vi "Get panel triangle edge link indices.vi"(1 "Panel triangles in":T1[](array[typedef])) -> (0 "Panel triangles out":T1[](array[typedef]))   [LabVIEW 2017]
uses:
  ctls/Triangle panel.ctl
  Dot product_3Dpf.vi
panel:
  out "Progress":i32(slide) scale=0.0..3330.0
  out "N panels":i32
  out "Panel number":i32
  # "Computing panel links (needed for sfc. gradient & Cp calcs.)"
  # "of"
  # "PN 23/10/17"
  # "Vertices"
  # "Edges"
  # "Unit normal"
  # "Control point"
  # "Edge\nlinks \n(tri index)"
  # "Vertices"
  # "Edges"
  # "Unit normal"
  # "Control point"
  # "Edge\nlinks \n(tri index)"
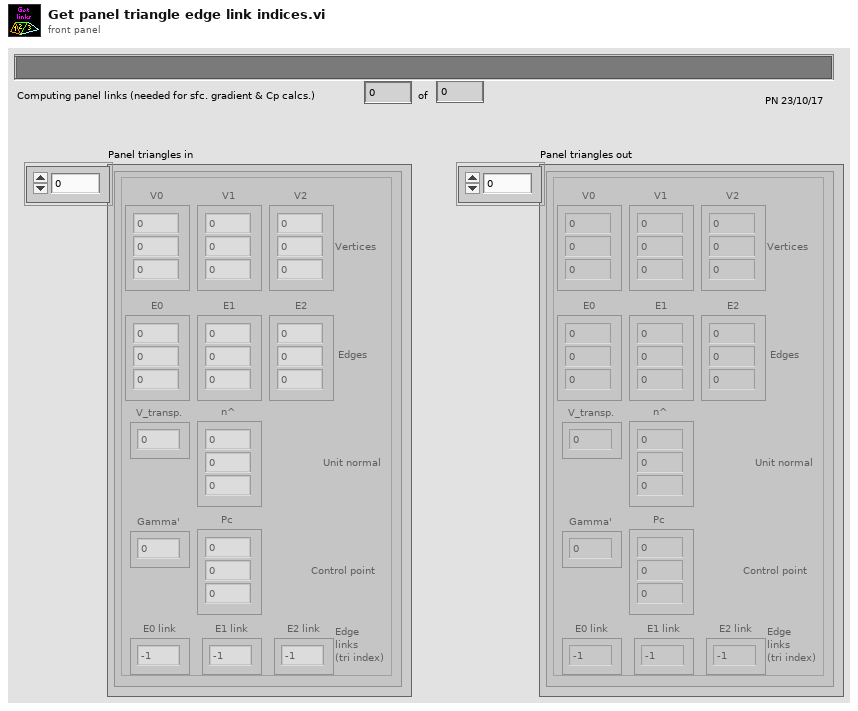
[diagram p1: front panel]
types:
  T1 = typedef "Triangle panel.ctl" = cluster{"V0":sgl[], "V1":sgl[], "V2":sgl[], "E0":sgl[], "E1":sgl[], "E2":sgl[], "n^":sgl[], "Pc":sgl[], "Gamma'":sgl, "V_transp.":sgl, "E0 link":i32, "E1 link":i32, "E2 link":i32}
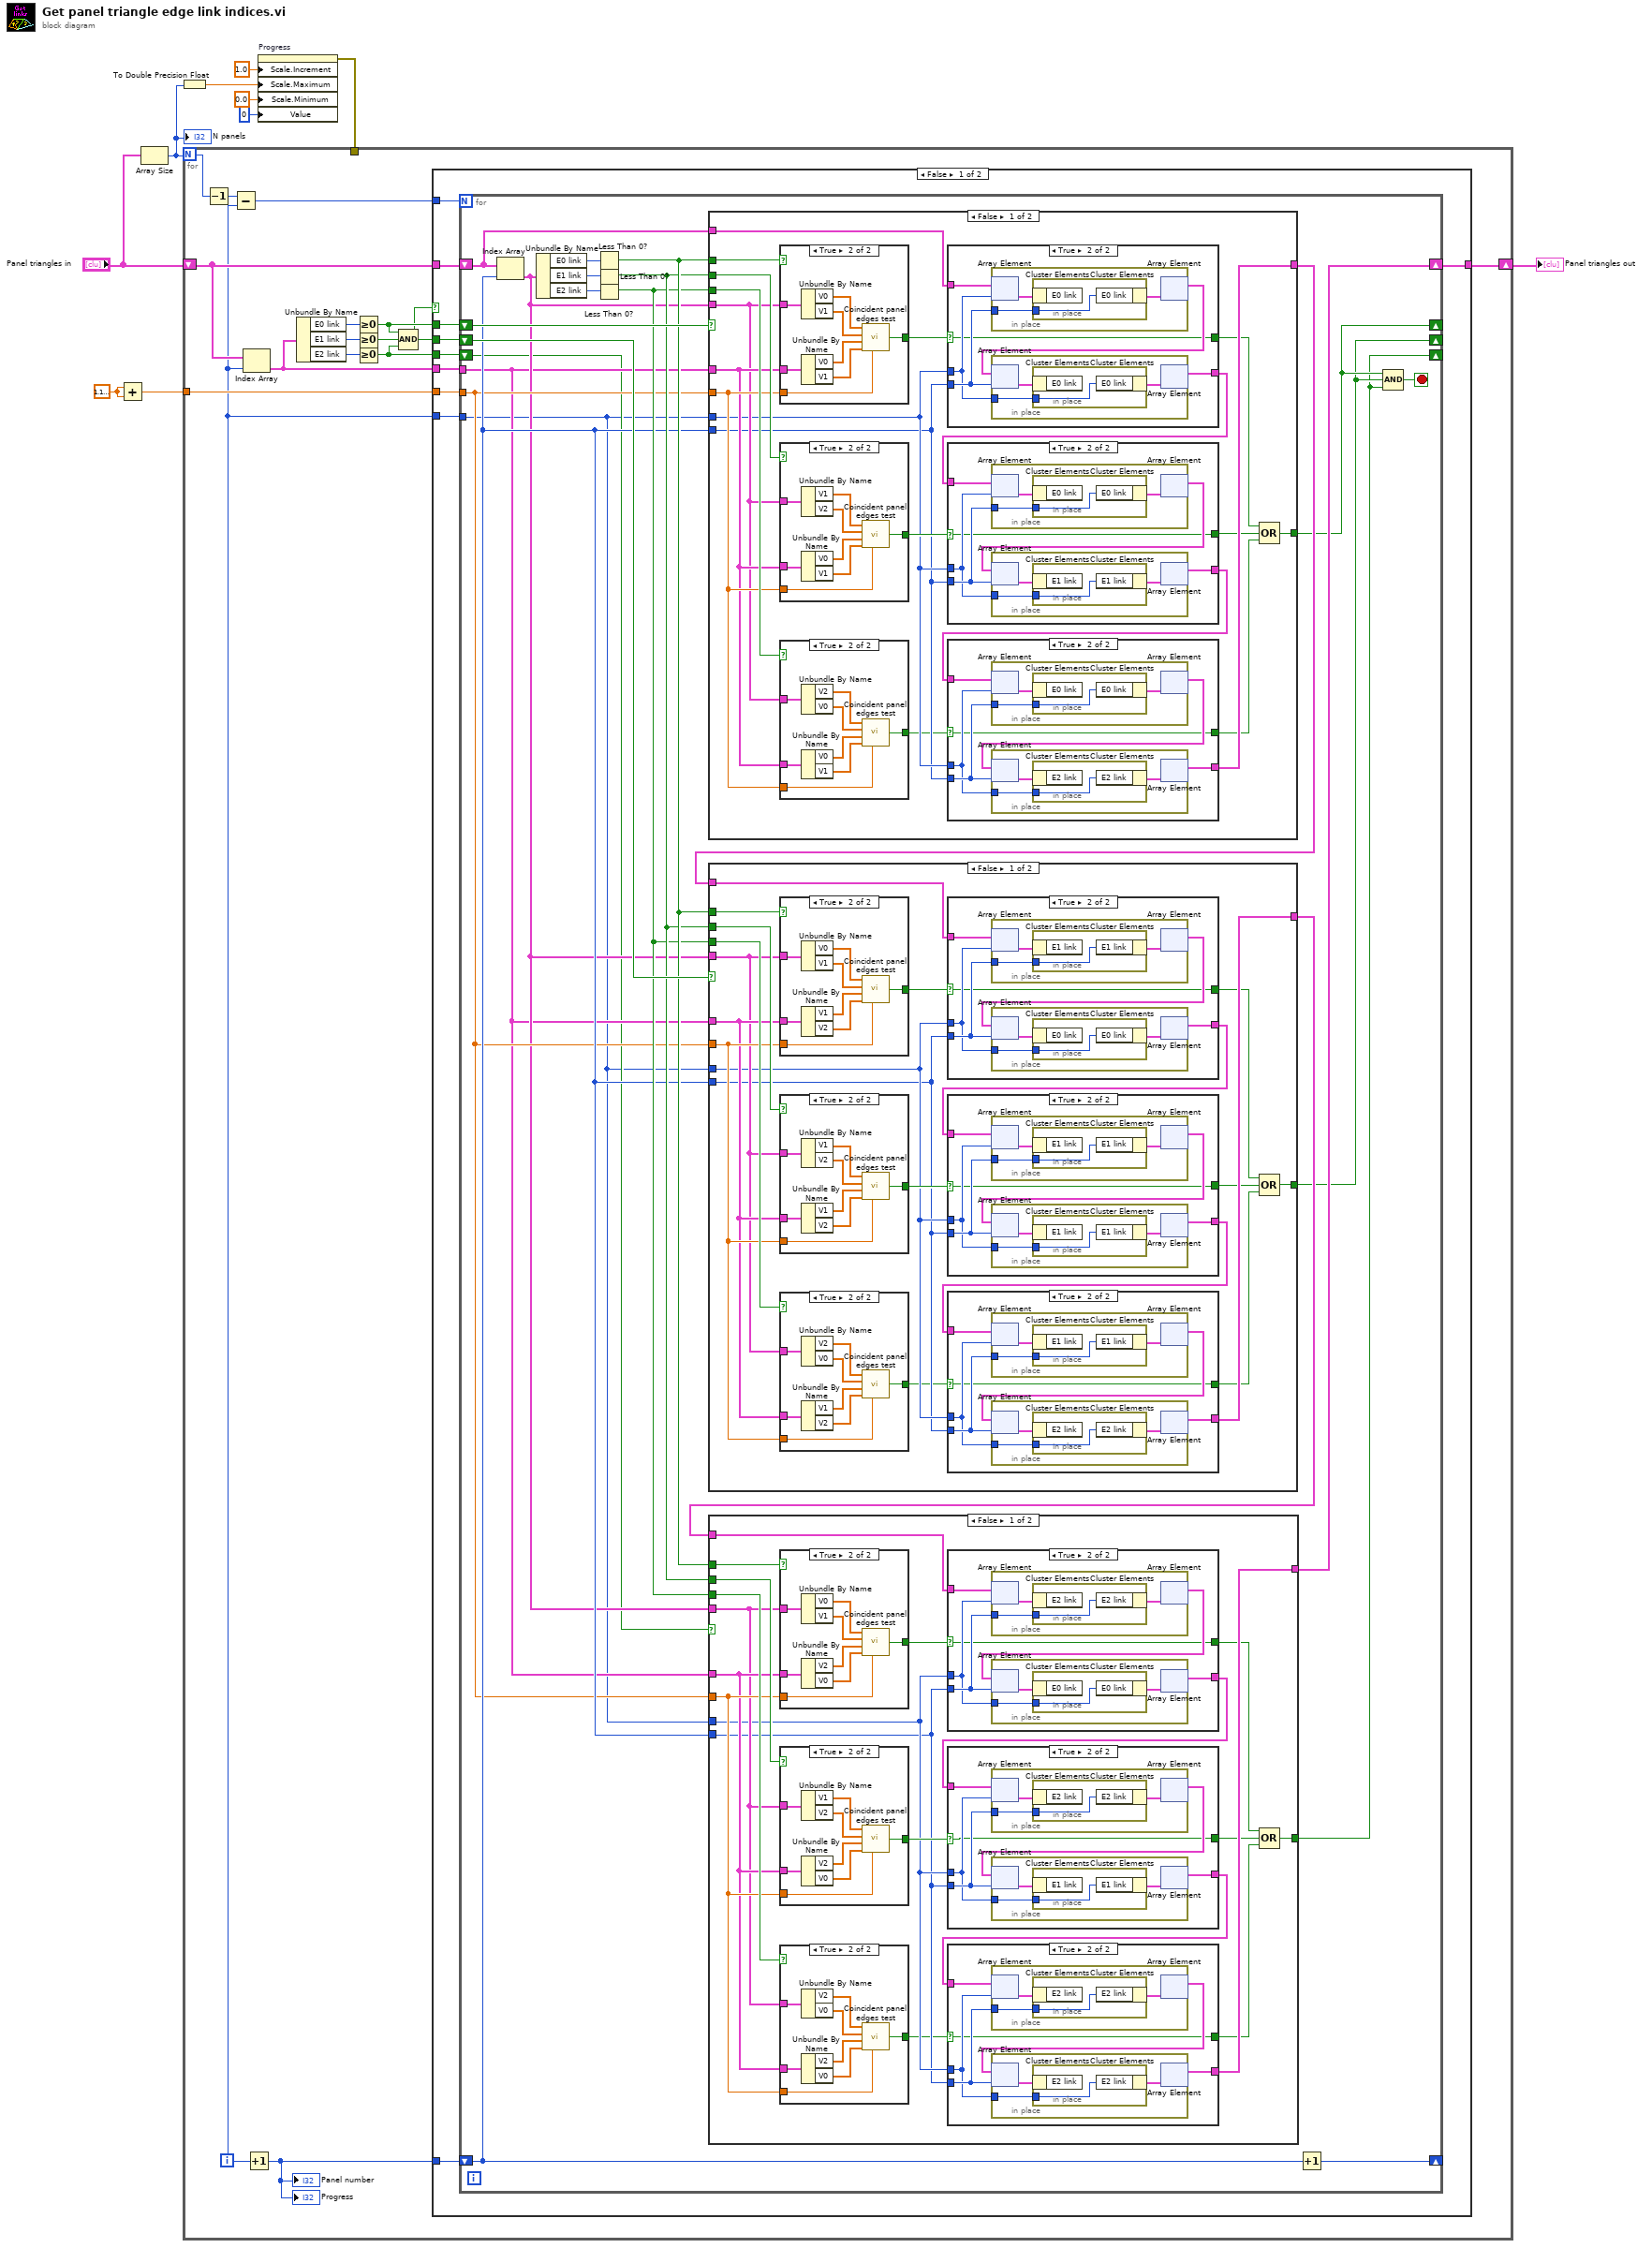
[diagram p0: block diagram]
diagram:
  w2 = sgl 1.1920929e-07
  n1 = Add(x=w2, y=w2) -> (x+y=w3:sgl)
  n2 = Array Size(array="Panel triangles in") -> (size(s)=w6:i32)
  "N panels" <- w6
  n3 = To Double Precision Float(number=w6) -> (double precision float=w1:dbl)
  n4 = property on="Progress" class="Slide (strict)"("Scale.Increment"=1.0 ("Scale.Range:Increment"), "Scale.Maximum"=w1, "Scale.Minimum"=0.0 ("Scale.Range:Minimum"), "Value"=0 ("Progress")) -> (error out=w4:errorcluster)  [unwired: 2 in, 1 out]
  n5 = for {
    N: w6 -> [w26]
    shift-right: [w12] -> w9
    shift-left: "Panel triangles in" -> [w16]
    tunnel: w3 -> [w14]
    tunnel: w4 -> [_]
    i -> [w13]
    n6 = Decrement(x=w26) -> (x-1=w25:i32)
    n7 = Subtract(x=w25, y=w13) -> (x-y=w24:i32)
    n8 = Index Array(array=w16, index=w13) -> (element=w15:T1)
    n9 = Increment(x=w13) -> (x+1=w11:i32)
    "Panel number" <- w11
    "Progress" <- w11
    n10 = Unbundle By Name(w15) -> ("E0 link"=w21:i32, "E1 link"=w22:i32, "E2 link"=w23:i32)
    n11 = Greater Or Equal To 0?(x=w21) -> (x >= 0?=w20:bool)
    n12 = Greater Or Equal To 0?(x=w22) -> (x >= 0?=w19:bool)
    n13 = Greater Or Equal To 0?(x=w23) -> (x >= 0?=w18:bool)
    n14 = Compound Arithmetic op=AND(w20, w19, w18) -> (w17:bool)
    n15 = case shown="False" w17 {
      tunnel: w24 -> [w36 _]
      tunnel: w11 -> [w35 _]
      tunnel: w16 -> [w34 w348]
      tunnel: w20 -> [w33 _]
      tunnel: w19 -> [w32 _]
      tunnel: w18 -> [w31 _]
      tunnel: w15 -> [w30 _]
      tunnel: w14 -> [w29 _]
      tunnel: w13 -> [w28 _]
      tunnel: [w27 w348] -> w12
      frame False {
        n16 = for {
          N: w36 -> [_]
          shift-right: [w59] -> _
          shift-left: w35 -> [w49]
          tunnel: w30 -> [w46]
          shift-right: [w44] -> w27
          shift-left: w34 -> [w53]
          tunnel: w29 -> [w48]
          tunnel: w28 -> [w43]
          shift-right: [w39] -> _
          shift-left: w33 -> [w55]
          shift-right: [w38] -> _
          shift-left: w32 -> [w54]
          shift-right: [w37] -> _
          shift-left: w31 -> [w45]
          stop <- w42 stop-if-true
          n17 = Index Array(array=w53, index=w49) -> (element=w47:T1)
          n18 = Unbundle By Name(w47) -> ("E0 link"=w56:i32, "E1 link"=w57:i32, "E2 link"=w58:i32)
          n19 = Less Than 0?(x=w56) -> (x < 0?=w52:bool)
          n20 = Less Than 0?(x=w57) -> (x < 0?=w51:bool)
          n21 = Less Than 0?(x=w58) -> (x < 0?=w50:bool)
          n22 = case shown="False" w55 {
            selector: w55 -> [_ w346]
            tunnel: w52 -> [w270 _]
            tunnel: w51 -> [w269 _]
            tunnel: w50 -> [w268 _]
            tunnel: w47 -> [w265 _]
            tunnel: w46 -> [w266 _]
            tunnel: w48 -> [w267 _]
            tunnel: w53 -> [w263 w347]
            tunnel: w43 -> [w259 _]
            tunnel: w49 -> [w258 _]
            tunnel: [w256 w347] -> w41
            tunnel: [w252 w346] -> w39
            frame False {
              n23 = case shown="True" w270 {
                selector: w270 -> [w337 _]
                tunnel: w265 -> [_ w345]
                tunnel: w266 -> [_ w344]
                tunnel: w267 -> [_ w339]
                tunnel: [w337 w338] -> w264
                frame False {
                }
                frame True {
                  n24 = Unbundle By Name(w345) -> ("V0"=w343:sgl[], "V1"=w342:sgl[])
                  n25 = Unbundle By Name(w344) -> ("V0"=w341:sgl[], "V1"=w340:sgl[])
                  n26 = call "Coincident panel edges test.vi"("epsilon"=w339, "V1_1"=w340, "V1_0"=w341, "V0_1"=w342, "V0_0"=w343) -> ("Edges are coincident"=w338:bool)  [unwired: 1 in]
                }
              }
              n27 = case shown="True" w269 {
                selector: w269 -> [w328 _]
                tunnel: w265 -> [_ w336]
                tunnel: w266 -> [_ w335]
                tunnel: w267 -> [_ w330]
                tunnel: [w328 w329] -> w261
                frame False {
                }
                frame True {
                  n28 = Unbundle By Name(w336) -> ("V1"=w334:sgl[], "V2"=w333:sgl[])
                  n29 = Unbundle By Name(w335) -> ("V0"=w332:sgl[], "V1"=w331:sgl[])
                  n30 = call "Coincident panel edges test.vi"("epsilon"=w330, "V1_1"=w331, "V1_0"=w332, "V0_1"=w333, "V0_0"=w334) -> ("Edges are coincident"=w329:bool)  [unwired: 1 in]
                }
              }
              n31 = case shown="True" w268 {
                selector: w268 -> [w319 _]
                tunnel: w265 -> [_ w327]
                tunnel: w266 -> [_ w326]
                tunnel: w267 -> [_ w321]
                tunnel: [w319 w320] -> w257
                frame False {
                }
                frame True {
                  n32 = Unbundle By Name(w327) -> ("V2"=w325:sgl[], "V0"=w324:sgl[])
                  n33 = Unbundle By Name(w326) -> ("V0"=w323:sgl[], "V1"=w322:sgl[])
                  n34 = call "Coincident panel edges test.vi"("epsilon"=w321, "V1_1"=w322, "V1_0"=w323, "V0_1"=w324, "V0_0"=w325) -> ("Edges are coincident"=w320:bool)  [unwired: 1 in]
                }
              }
              n35 = case shown="True" w264 {
                selector: w264 -> [w303 w305]
                tunnel: w263 -> [w304 w310]
                tunnel: w259 -> [_ w307]
                tunnel: w258 -> [_ w308]
                tunnel: [w304 w306] -> w262
                tunnel: [w303 w305] -> w254
                frame False {
                }
                frame True {
                  n36 = in-place {
                    in-place-border: w308 -> [w316]
                    n37 = in-place-array #1(w310, w307) -> (w317:T1)
                    n38 = in-place {
                      in-place-border: w316 -> [w318]
                      n39 = in-place-cluster #2(w317) -> ()  [unwired: 1 out]
                      n40 = in-place-cluster #2("E0 link"=w318) -> (w315:T1)
                    }
                    n41 = in-place-array #1(w315) -> (w309:T1[])  [unwired: 1 out]
                  }
                  n42 = in-place {
                    in-place-border: w307 -> [w312]
                    n43 = in-place-array #3(w309, w308) -> (w313:T1)
                    n44 = in-place {
                      in-place-border: w312 -> [w314]
                      n45 = in-place-cluster #4(w313) -> ()  [unwired: 1 out]
                      n46 = in-place-cluster #4("E0 link"=w314) -> (w311:T1)
                    }
                    n47 = in-place-array #3(w311) -> (w306:T1[])  [unwired: 1 out]
                  }
                }
              }
              n48 = case shown="True" w261 {
                selector: w261 -> [w287 w289]
                tunnel: w262 -> [w288 w294]
                tunnel: w259 -> [_ w291]
                tunnel: w258 -> [_ w292]
                tunnel: [w288 w290] -> w260
                tunnel: [w287 w289] -> w255
                frame False {
                }
                frame True {
                  n49 = in-place {
                    in-place-border: w292 -> [w300]
                    n50 = in-place-array #5(w294, w291) -> (w301:T1)
                    n51 = in-place {
                      in-place-border: w300 -> [w302]
                      n52 = in-place-cluster #6(w301) -> ()  [unwired: 1 out]
                      n53 = in-place-cluster #6("E0 link"=w302) -> (w299:T1)
                    }
                    n54 = in-place-array #5(w299) -> (w293:T1[])  [unwired: 1 out]
                  }
                  n55 = in-place {
                    in-place-border: w291 -> [w296]
                    n56 = in-place-array #7(w293, w292) -> (w297:T1)
                    n57 = in-place {
                      in-place-border: w296 -> [w298]
                      n58 = in-place-cluster #8(w297) -> ()  [unwired: 1 out]
                      n59 = in-place-cluster #8("E1 link"=w298) -> (w295:T1)
                    }
                    n60 = in-place-array #7(w295) -> (w290:T1[])  [unwired: 1 out]
                  }
                }
              }
              n61 = case shown="True" w257 {
                selector: w257 -> [w271 w273]
                tunnel: w260 -> [w272 w278]
                tunnel: w259 -> [_ w275]
                tunnel: w258 -> [_ w276]
                tunnel: [w272 w274] -> w256
                tunnel: [w271 w273] -> w253
                frame False {
                }
                frame True {
                  n62 = in-place {
                    in-place-border: w276 -> [w284]
                    n63 = in-place-array #9(w278, w275) -> (w285:T1)
                    n64 = in-place {
                      in-place-border: w284 -> [w286]
                      n65 = in-place-cluster #10(w285) -> ()  [unwired: 1 out]
                      n66 = in-place-cluster #10("E0 link"=w286) -> (w283:T1)
                    }
                    n67 = in-place-array #9(w283) -> (w277:T1[])  [unwired: 1 out]
                  }
                  n68 = in-place {
                    in-place-border: w275 -> [w280]
                    n69 = in-place-array #11(w277, w276) -> (w281:T1)
                    n70 = in-place {
                      in-place-border: w280 -> [w282]
                      n71 = in-place-cluster #12(w281) -> ()  [unwired: 1 out]
                      n72 = in-place-cluster #12("E2 link"=w282) -> (w279:T1)
                    }
                    n73 = in-place-array #11(w279) -> (w274:T1[])  [unwired: 1 out]
                  }
                }
              }
              n74 = Compound Arithmetic op=OR(w254, w255, w253) -> (w252:bool)
            }
            frame True {
            }
          }
          n75 = case shown="False" w54 {
            selector: w54 -> [_ w250]
            tunnel: w52 -> [w174 _]
            tunnel: w51 -> [w173 _]
            tunnel: w50 -> [w172 _]
            tunnel: w47 -> [w169 _]
            tunnel: w46 -> [w170 _]
            tunnel: w48 -> [w171 _]
            tunnel: w41 -> [w167 w251]
            tunnel: w43 -> [w163 _]
            tunnel: w49 -> [w162 _]
            tunnel: [w160 w251] -> w40
            tunnel: [w156 w250] -> w38
            frame False {
              n76 = case shown="True" w174 {
                selector: w174 -> [w241 _]
                tunnel: w169 -> [_ w249]
                tunnel: w170 -> [_ w248]
                tunnel: w171 -> [_ w243]
                tunnel: [w241 w242] -> w168
                frame False {
                }
                frame True {
                  n77 = Unbundle By Name(w249) -> ("V0"=w247:sgl[], "V1"=w246:sgl[])
                  n78 = Unbundle By Name(w248) -> ("V1"=w245:sgl[], "V2"=w244:sgl[])
                  n79 = call "Coincident panel edges test.vi"("epsilon"=w243, "V1_1"=w244, "V1_0"=w245, "V0_1"=w246, "V0_0"=w247) -> ("Edges are coincident"=w242:bool)  [unwired: 1 in]
                }
              }
              n80 = case shown="True" w173 {
                selector: w173 -> [w232 _]
                tunnel: w169 -> [_ w240]
                tunnel: w170 -> [_ w239]
                tunnel: w171 -> [_ w234]
                tunnel: [w232 w233] -> w165
                frame False {
                }
                frame True {
                  n81 = Unbundle By Name(w240) -> ("V1"=w238:sgl[], "V2"=w237:sgl[])
                  n82 = Unbundle By Name(w239) -> ("V1"=w236:sgl[], "V2"=w235:sgl[])
                  n83 = call "Coincident panel edges test.vi"("epsilon"=w234, "V1_1"=w235, "V1_0"=w236, "V0_1"=w237, "V0_0"=w238) -> ("Edges are coincident"=w233:bool)  [unwired: 1 in]
                }
              }
              n84 = case shown="True" w172 {
                selector: w172 -> [w223 _]
                tunnel: w169 -> [_ w231]
                tunnel: w170 -> [_ w230]
                tunnel: w171 -> [_ w225]
                tunnel: [w223 w224] -> w161
                frame False {
                }
                frame True {
                  n85 = Unbundle By Name(w231) -> ("V2"=w229:sgl[], "V0"=w228:sgl[])
                  n86 = Unbundle By Name(w230) -> ("V1"=w227:sgl[], "V2"=w226:sgl[])
                  n87 = call "Coincident panel edges test.vi"("epsilon"=w225, "V1_1"=w226, "V1_0"=w227, "V0_1"=w228, "V0_0"=w229) -> ("Edges are coincident"=w224:bool)  [unwired: 1 in]
                }
              }
              n88 = case shown="True" w168 {
                selector: w168 -> [w207 w209]
                tunnel: w167 -> [w208 w214]
                tunnel: w163 -> [_ w211]
                tunnel: w162 -> [_ w212]
                tunnel: [w208 w210] -> w166
                tunnel: [w207 w209] -> w158
                frame False {
                }
                frame True {
                  n89 = in-place {
                    in-place-border: w212 -> [w220]
                    n90 = in-place-array #13(w214, w211) -> (w221:T1)
                    n91 = in-place {
                      in-place-border: w220 -> [w222]
                      n92 = in-place-cluster #14(w221) -> ()  [unwired: 1 out]
                      n93 = in-place-cluster #14("E1 link"=w222) -> (w219:T1)
                    }
                    n94 = in-place-array #13(w219) -> (w213:T1[])  [unwired: 1 out]
                  }
                  n95 = in-place {
                    in-place-border: w211 -> [w216]
                    n96 = in-place-array #15(w213, w212) -> (w217:T1)
                    n97 = in-place {
                      in-place-border: w216 -> [w218]
                      n98 = in-place-cluster #16(w217) -> ()  [unwired: 1 out]
                      n99 = in-place-cluster #16("E0 link"=w218) -> (w215:T1)
                    }
                    n100 = in-place-array #15(w215) -> (w210:T1[])  [unwired: 1 out]
                  }
                }
              }
              n101 = case shown="True" w165 {
                selector: w165 -> [w191 w193]
                tunnel: w166 -> [w192 w198]
                tunnel: w163 -> [_ w195]
                tunnel: w162 -> [_ w196]
                tunnel: [w192 w194] -> w164
                tunnel: [w191 w193] -> w159
                frame False {
                }
                frame True {
                  n102 = in-place {
                    in-place-border: w196 -> [w204]
                    n103 = in-place-array #17(w198, w195) -> (w205:T1)
                    n104 = in-place {
                      in-place-border: w204 -> [w206]
                      n105 = in-place-cluster #18(w205) -> ()  [unwired: 1 out]
                      n106 = in-place-cluster #18("E1 link"=w206) -> (w203:T1)
                    }
                    n107 = in-place-array #17(w203) -> (w197:T1[])  [unwired: 1 out]
                  }
                  n108 = in-place {
                    in-place-border: w195 -> [w200]
                    n109 = in-place-array #19(w197, w196) -> (w201:T1)
                    n110 = in-place {
                      in-place-border: w200 -> [w202]
                      n111 = in-place-cluster #20(w201) -> ()  [unwired: 1 out]
                      n112 = in-place-cluster #20("E1 link"=w202) -> (w199:T1)
                    }
                    n113 = in-place-array #19(w199) -> (w194:T1[])  [unwired: 1 out]
                  }
                }
              }
              n114 = case shown="True" w161 {
                selector: w161 -> [w175 w177]
                tunnel: w164 -> [w176 w182]
                tunnel: w163 -> [_ w179]
                tunnel: w162 -> [_ w180]
                tunnel: [w176 w178] -> w160
                tunnel: [w175 w177] -> w157
                frame False {
                }
                frame True {
                  n115 = in-place {
                    in-place-border: w180 -> [w188]
                    n116 = in-place-array #21(w182, w179) -> (w189:T1)
                    n117 = in-place {
                      in-place-border: w188 -> [w190]
                      n118 = in-place-cluster #22(w189) -> ()  [unwired: 1 out]
                      n119 = in-place-cluster #22("E1 link"=w190) -> (w187:T1)
                    }
                    n120 = in-place-array #21(w187) -> (w181:T1[])  [unwired: 1 out]
                  }
                  n121 = in-place {
                    in-place-border: w179 -> [w184]
                    n122 = in-place-array #23(w181, w180) -> (w185:T1)
                    n123 = in-place {
                      in-place-border: w184 -> [w186]
                      n124 = in-place-cluster #24(w185) -> ()  [unwired: 1 out]
                      n125 = in-place-cluster #24("E2 link"=w186) -> (w183:T1)
                    }
                    n126 = in-place-array #23(w183) -> (w178:T1[])  [unwired: 1 out]
                  }
                }
              }
              n127 = Compound Arithmetic op=OR(w158, w159, w157) -> (w156:bool)
            }
            frame True {
            }
          }
          n128 = case shown="False" w45 {
            selector: w45 -> [_ w154]
            tunnel: w52 -> [w78 _]
            tunnel: w51 -> [w77 _]
            tunnel: w50 -> [w76 _]
            tunnel: w47 -> [w73 _]
            tunnel: w46 -> [w74 _]
            tunnel: w48 -> [w75 _]
            tunnel: w40 -> [w71 w155]
            tunnel: w43 -> [w67 _]
            tunnel: w49 -> [w66 _]
            tunnel: [w64 w155] -> w44
            tunnel: [w60 w154] -> w37
            frame False {
              n129 = case shown="True" w78 {
                selector: w78 -> [w145 _]
                tunnel: w73 -> [_ w153]
                tunnel: w74 -> [_ w152]
                tunnel: w75 -> [_ w147]
                tunnel: [w145 w146] -> w72
                frame False {
                }
                frame True {
                  n130 = Unbundle By Name(w153) -> ("V0"=w151:sgl[], "V1"=w150:sgl[])
                  n131 = Unbundle By Name(w152) -> ("V2"=w149:sgl[], "V0"=w148:sgl[])
                  n132 = call "Coincident panel edges test.vi"("epsilon"=w147, "V1_1"=w148, "V1_0"=w149, "V0_1"=w150, "V0_0"=w151) -> ("Edges are coincident"=w146:bool)  [unwired: 1 in]
                }
              }
              n133 = case shown="True" w77 {
                selector: w77 -> [w136 _]
                tunnel: w73 -> [_ w144]
                tunnel: w74 -> [_ w143]
                tunnel: w75 -> [_ w138]
                tunnel: [w136 w137] -> w69
                frame False {
                }
                frame True {
                  n134 = Unbundle By Name(w144) -> ("V1"=w142:sgl[], "V2"=w141:sgl[])
                  n135 = Unbundle By Name(w143) -> ("V2"=w140:sgl[], "V0"=w139:sgl[])
                  n136 = call "Coincident panel edges test.vi"("epsilon"=w138, "V1_1"=w139, "V1_0"=w140, "V0_1"=w141, "V0_0"=w142) -> ("Edges are coincident"=w137:bool)  [unwired: 1 in]
                }
              }
              n137 = case shown="True" w76 {
                selector: w76 -> [w127 _]
                tunnel: w73 -> [_ w135]
                tunnel: w74 -> [_ w134]
                tunnel: w75 -> [_ w129]
                tunnel: [w127 w128] -> w65
                frame False {
                }
                frame True {
                  n138 = Unbundle By Name(w135) -> ("V2"=w133:sgl[], "V0"=w132:sgl[])
                  n139 = Unbundle By Name(w134) -> ("V2"=w131:sgl[], "V0"=w130:sgl[])
                  n140 = call "Coincident panel edges test.vi"("epsilon"=w129, "V1_1"=w130, "V1_0"=w131, "V0_1"=w132, "V0_0"=w133) -> ("Edges are coincident"=w128:bool)  [unwired: 1 in]
                }
              }
              n141 = case shown="True" w72 {
                selector: w72 -> [w111 w113]
                tunnel: w71 -> [w112 w118]
                tunnel: w67 -> [_ w115]
                tunnel: w66 -> [_ w116]
                tunnel: [w112 w114] -> w70
                tunnel: [w111 w113] -> w62
                frame False {
                }
                frame True {
                  n142 = in-place {
                    in-place-border: w116 -> [w124]
                    n143 = in-place-array #25(w118, w115) -> (w125:T1)
                    n144 = in-place {
                      in-place-border: w124 -> [w126]
                      n145 = in-place-cluster #26(w125) -> ()  [unwired: 1 out]
                      n146 = in-place-cluster #26("E2 link"=w126) -> (w123:T1)
                    }
                    n147 = in-place-array #25(w123) -> (w117:T1[])  [unwired: 1 out]
                  }
                  n148 = in-place {
                    in-place-border: w115 -> [w120]
                    n149 = in-place-array #27(w117, w116) -> (w121:T1)
                    n150 = in-place {
                      in-place-border: w120 -> [w122]
                      n151 = in-place-cluster #28(w121) -> ()  [unwired: 1 out]
                      n152 = in-place-cluster #28("E0 link"=w122) -> (w119:T1)
                    }
                    n153 = in-place-array #27(w119) -> (w114:T1[])  [unwired: 1 out]
                  }
                }
              }
              n154 = case shown="True" w69 {
                selector: w69 -> [w95 w97]
                tunnel: w70 -> [w96 w102]
                tunnel: w67 -> [_ w99]
                tunnel: w66 -> [_ w100]
                tunnel: [w96 w98] -> w68
                tunnel: [w95 w97] -> w63
                frame False {
                }
                frame True {
                  n155 = in-place {
                    in-place-border: w100 -> [w108]
                    n156 = in-place-array #29(w102, w99) -> (w109:T1)
                    n157 = in-place {
                      in-place-border: w108 -> [w110]
                      n158 = in-place-cluster #30(w109) -> ()  [unwired: 1 out]
                      n159 = in-place-cluster #30("E2 link"=w110) -> (w107:T1)
                    }
                    n160 = in-place-array #29(w107) -> (w101:T1[])  [unwired: 1 out]
                  }
                  n161 = in-place {
                    in-place-border: w99 -> [w104]
                    n162 = in-place-array #31(w101, w100) -> (w105:T1)
                    n163 = in-place {
                      in-place-border: w104 -> [w106]
                      n164 = in-place-cluster #32(w105) -> ()  [unwired: 1 out]
                      n165 = in-place-cluster #32("E1 link"=w106) -> (w103:T1)
                    }
                    n166 = in-place-array #31(w103) -> (w98:T1[])  [unwired: 1 out]
                  }
                }
              }
              n167 = case shown="True" w65 {
                selector: w65 -> [w79 w81]
                tunnel: w68 -> [w80 w86]
                tunnel: w67 -> [_ w83]
                tunnel: w66 -> [_ w84]
                tunnel: [w80 w82] -> w64
                tunnel: [w79 w81] -> w61
                frame False {
                }
                frame True {
                  n168 = in-place {
                    in-place-border: w84 -> [w92]
                    n169 = in-place-array #33(w86, w83) -> (w93:T1)
                    n170 = in-place {
                      in-place-border: w92 -> [w94]
                      n171 = in-place-cluster #34(w93) -> ()  [unwired: 1 out]
                      n172 = in-place-cluster #34("E2 link"=w94) -> (w91:T1)
                    }
                    n173 = in-place-array #33(w91) -> (w85:T1[])  [unwired: 1 out]
                  }
                  n174 = in-place {
                    in-place-border: w83 -> [w88]
                    n175 = in-place-array #35(w85, w84) -> (w89:T1)
                    n176 = in-place {
                      in-place-border: w88 -> [w90]
                      n177 = in-place-cluster #36(w89) -> ()  [unwired: 1 out]
                      n178 = in-place-cluster #36("E2 link"=w90) -> (w87:T1)
                    }
                    n179 = in-place-array #35(w87) -> (w82:T1[])  [unwired: 1 out]
                  }
                }
              }
              n180 = Compound Arithmetic op=OR(w62, w63, w61) -> (w60:bool)
            }
            frame True {
            }
          }
          n181 = Increment(x=w49) -> (x+1=w59:i32)
          n182 = Compound Arithmetic op=AND(w39, w38, w37) -> (w42:bool)
        }
      }
      frame True {
      }
    }
  }
  "Panel triangles out" <- w9
